vi "Execute Filling.vi"(8 "error in":errorcluster, 11 "CPC in":refnum<class "CPC.lvclass">) -> (0 "error out":errorcluster, 2 "CMD Good":bool, 3 "CPC out":refnum<class "CPC.lvclass">)   [LabVIEW 2014, in "CPC.lvclass"]
uses:
  CPC.lvclass
  CPC.lvclass/CPC.ctl
  reusable/Session APIs/Serial/Public/Get Data/Get String.vi
  reusable/Session APIs/Serial/Serial Session.lvclass
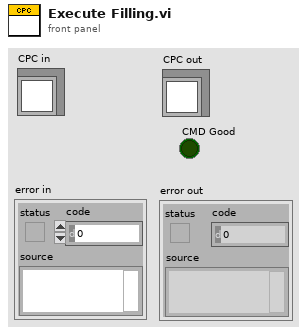
[diagram p1: front panel]
types:
  T1 = typedef "Serial Session.lvclass/Session Handle.ctl" = refnum<data-value>
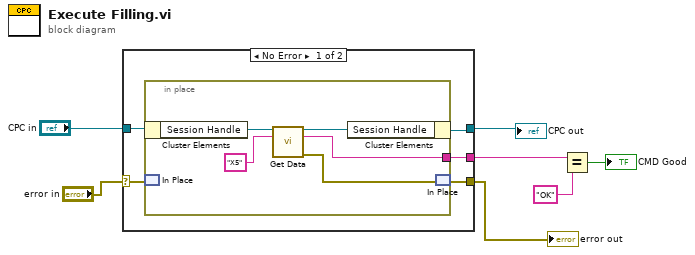
[diagram p0: block diagram]
diagram:
  n1 = case shown="No Error" "error in" {
    selector: "error in" -> [w11 w19]
    tunnel: "CPC in" -> [w12 w18]
    tunnel: [w9 w19] -> w2
    tunnel: [w10 w18] -> w3
    tunnel: [w8 _] -> w4
    frame No Error {
      n2 = in-place {
        in-place-border: [w13] -> w8
        n3 = in-place-cluster #1(w12) -> ("Session Handle"=w17:T1)
        n4 = in-place-match #2(w11) -> ()  [unwired: 1 out]
        n5 = call-poly "Get Data.vi"("Session Handle in"=w17, "CMD"="X5" ("string")) -> ("Session Handle out"=w16:T1, "DataOut"=w13:string, "error out"=w14:errorcluster)  [unwired: 11 in]
        n6 = in-place-cluster #1("Session Handle"=w16) -> (w10:refnum<class "CPC.lvclass">)
        n7 = in-place-match #2(w14) -> (w9:errorcluster)
      }
    }
    frame Error {
    }
  }
  "error out" <- w2
  "CPC out" <- w3
  n8 = Equal?(x=w4, y="OK") -> (x = y?=→"CMD Good":bool)
